vi "Tube Select.vi"(8 "error in (no error)":errorcluster) -> (0 "error out":errorcluster, 1 "Close":bool, 2 "Load":bool, 3 "SelectedTube":i32)   [LabVIEW 2023]
panel:
  in  "Close":bool
  in  "TubeSel":T1
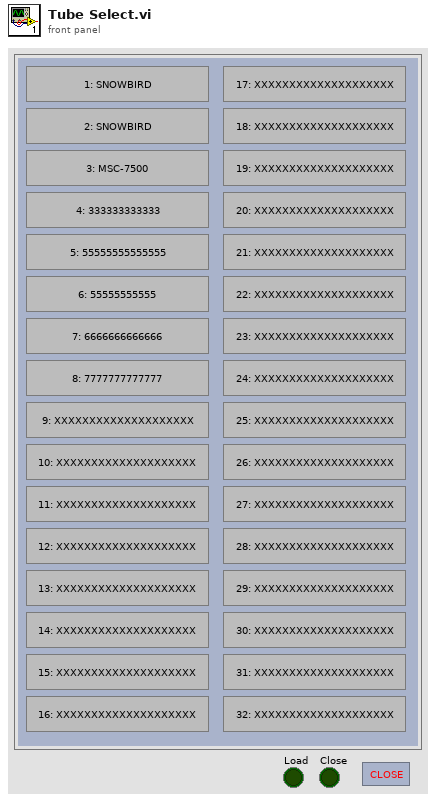
[diagram p1: front panel]
types:
  T1 = cluster{"OK Button 1":bool, "OK Button 2":bool, "OK Button 3":bool, "OK Button 4":bool, "OK Button 5":bool, "OK Button 6":bool, "OK Button 7":bool, "OK Button 8":bool, "OK Button 9":bool, "OK Button 10":bool, "OK Button 11":bool, "OK Button 12":bool, "OK Button 13":bool, "OK Button 14":bool, "OK Button 15":bool, "OK Button 16":bool, "OK Button 17":bool, "OK Button 18":bool, "OK Button 19":bool, "OK Button 20":bool, "OK Button 21":bool, "OK Button 22":bool, "OK Button 23":bool, "OK Button 24":bool, "OK Button 25":bool, "OK Button 26":bool, "OK Button 27":bool, "OK Button 28":bool, "OK Button 29":bool, "OK Button 30":bool, "OK Button 31":bool, "OK Button 32":bool}
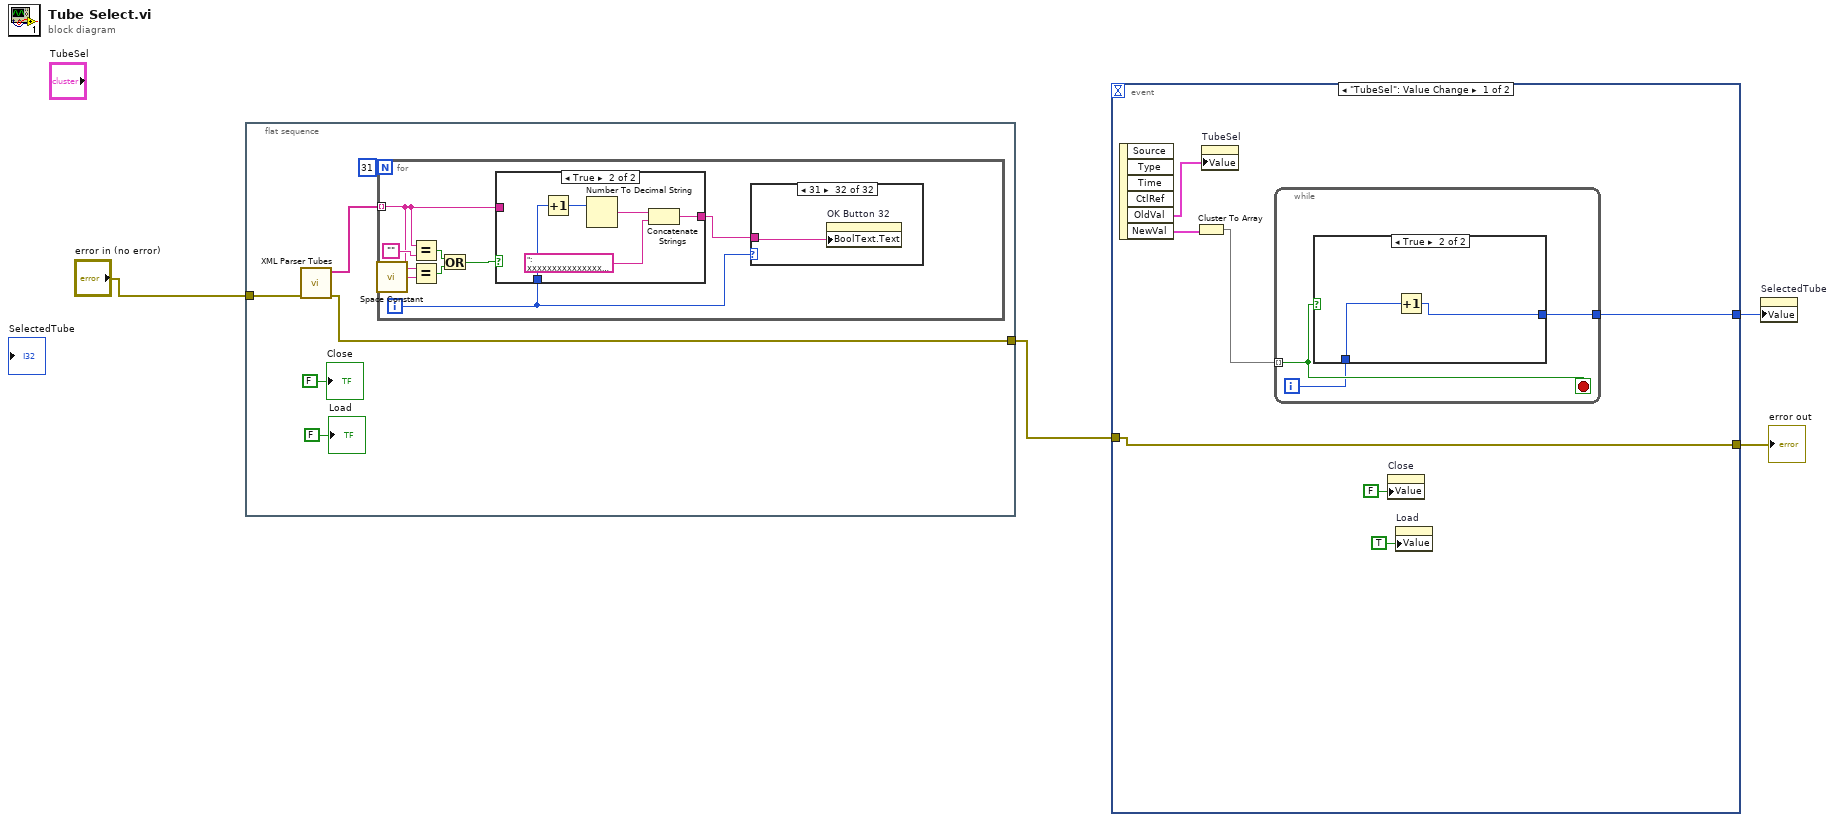
[diagram p0: block diagram]
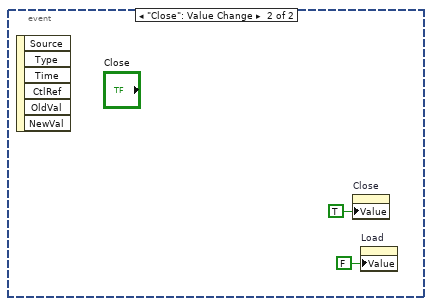
[diagram p3: hidden frame]
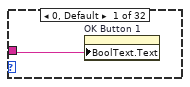
[diagram p4: hidden frame]
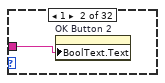
[diagram p5: hidden frame]
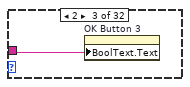
[diagram p6: hidden frame]
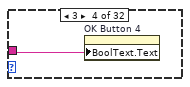
[diagram p7: hidden frame]
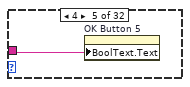
[diagram p8: hidden frame]
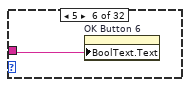
[diagram p9: hidden frame]
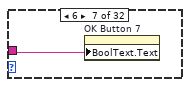
[diagram p10: hidden frame]
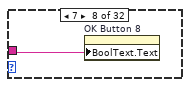
[diagram p11: hidden frame]
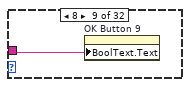
[diagram p12: hidden frame]
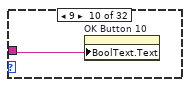
[diagram p13: hidden frame]
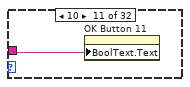
[diagram p14: hidden frame]
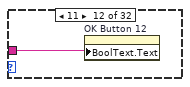
[diagram p15: hidden frame]
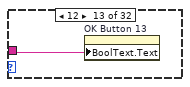
[diagram p16: hidden frame]
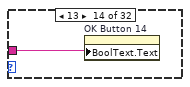
[diagram p17: hidden frame]
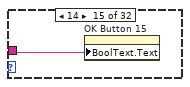
[diagram p18: hidden frame]
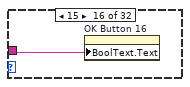
[diagram p19: hidden frame]
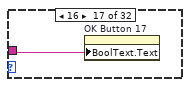
[diagram p20: hidden frame]
diagram:
  n1 = flat-sequence {
    tunnel: "error in (no error)" -> [w8]
    tunnel: [w7] -> w2
    frame #0 {
      n2 = call "XML Parser Tubes.vi"("error in (no error)"=w8) -> ("error out"=w7:errorcluster, "output array"=w10:string[])  [unwired: 9 in]
      n3 = for {
        N: 31 -> [_]
        tunnel: w10 -> [w13] mode=indexing
        i -> [w12]
        n4 = call <vilib>:"Space Constant.vi"() -> ("String"=w17:string)
        n5 = Equal?(x=w13, y="") -> (x = y?=w16:bool)
        n6 = Equal?(x=w13, y=w17) -> (x = y?=w15:bool)
        n7 = Or(x=w16, y=w15) -> (x .or. y?=w14:bool)
        n8 = case shown="True" w14 {
          tunnel: w13 -> [w54 _]
          tunnel: w12 -> [w51 w57]
          tunnel: [w53 w59] -> w11
          frame False {
            n9 = Increment(x=w51) -> (x+1=w52:i32)
            n10 = Number To Decimal String(number=w52) -> (decimal integer string=w56:string)  [unwired: 1 in]
            n11 = Concatenate Strings(w56, ": ", w54) -> (w53:string)
          }
          frame True {
            n12 = Increment(x=w57) -> (x+1=w58:i32)
            n13 = Number To Decimal String(number=w58) -> (decimal integer string=w61:string)  [unwired: 1 in]
            n14 = Concatenate Strings(w61, ": XXXXXXXXXXXXXXXXXXXX") -> (w59:string)
          }
        }
        n15 = case shown="31" w12 {
          tunnel: w11 -> [w19 w20 w21 w22 w23 w24 w25 w26 w27 w28 w29 w30 w31 w32 w33 w34 w35 w36 w37 w38 w39 w40 w41 w42 w43 w44 w45 w46 w47 w48 w49 w50]
          frame 0, Default {
            n16 = property on="OK Button 1" class="Bool (strict)"("BoolText.Text"=w19) -> ()  [unwired: 2 in, 2 out]
          }
          frame 1 {
            n17 = property on="OK Button 2" class="Bool (strict)"("BoolText.Text"=w20) -> ()  [unwired: 2 in, 2 out]
          }
          frame 2 {
            n18 = property on="OK Button 3" class="Bool (strict)"("BoolText.Text"=w21) -> ()  [unwired: 2 in, 2 out]
          }
          frame 3 {
            n19 = property on="OK Button 4" class="Bool (strict)"("BoolText.Text"=w22) -> ()  [unwired: 2 in, 2 out]
          }
          frame 4 {
            n20 = property on="OK Button 5" class="Bool (strict)"("BoolText.Text"=w23) -> ()  [unwired: 2 in, 2 out]
          }
          frame 5 {
            n21 = property on="OK Button 6" class="Bool (strict)"("BoolText.Text"=w24) -> ()  [unwired: 2 in, 2 out]
          }
          frame 6 {
            n22 = property on="OK Button 7" class="Bool (strict)"("BoolText.Text"=w25) -> ()  [unwired: 2 in, 2 out]
          }
          frame 7 {
            n23 = property on="OK Button 8" class="Bool (strict)"("BoolText.Text"=w26) -> ()  [unwired: 2 in, 2 out]
          }
          frame 8 {
            n24 = property on="OK Button 9" class="Bool (strict)"("BoolText.Text"=w27) -> ()  [unwired: 2 in, 2 out]
          }
          frame 9 {
            n25 = property on="OK Button 10" class="Bool (strict)"("BoolText.Text"=w28) -> ()  [unwired: 2 in, 2 out]
          }
          frame 10 {
            n26 = property on="OK Button 11" class="Bool (strict)"("BoolText.Text"=w29) -> ()  [unwired: 2 in, 2 out]
          }
          frame 11 {
            n27 = property on="OK Button 12" class="Bool (strict)"("BoolText.Text"=w30) -> ()  [unwired: 2 in, 2 out]
          }
          frame 12 {
            n28 = property on="OK Button 13" class="Bool (strict)"("BoolText.Text"=w31) -> ()  [unwired: 2 in, 2 out]
          }
          frame 13 {
            n29 = property on="OK Button 14" class="Bool (strict)"("BoolText.Text"=w32) -> ()  [unwired: 2 in, 2 out]
          }
          frame 14 {
            n30 = property on="OK Button 15" class="Bool (strict)"("BoolText.Text"=w33) -> ()  [unwired: 2 in, 2 out]
          }
          frame 15 {
            n31 = property on="OK Button 16" class="Bool (strict)"("BoolText.Text"=w34) -> ()  [unwired: 2 in, 2 out]
          }
          frame 16 {
            n32 = property on="OK Button 17" class="Bool (strict)"("BoolText.Text"=w35) -> ()  [unwired: 2 in, 2 out]
          }
          frame 17 {
            n33 = property on="OK Button 18" class="Bool (strict)"("BoolText.Text"=w36) -> ()  [unwired: 2 in, 2 out]
          }
          frame 18 {
            n34 = property on="OK Button 19" class="Bool (strict)"("BoolText.Text"=w37) -> ()  [unwired: 2 in, 2 out]
          }
          frame 19 {
            n35 = property on="OK Button 20" class="Bool (strict)"("BoolText.Text"=w38) -> ()  [unwired: 2 in, 2 out]
          }
          frame 20 {
            n36 = property on="OK Button 21" class="Bool (strict)"("BoolText.Text"=w39) -> ()  [unwired: 2 in, 2 out]
          }
          frame 21 {
            n37 = property on="OK Button 22" class="Bool (strict)"("BoolText.Text"=w40) -> ()  [unwired: 2 in, 2 out]
          }
          frame 22 {
            n38 = property on="OK Button 23" class="Bool (strict)"("BoolText.Text"=w41) -> ()  [unwired: 2 in, 2 out]
          }
          frame 23 {
            n39 = property on="OK Button 24" class="Bool (strict)"("BoolText.Text"=w42) -> ()  [unwired: 2 in, 2 out]
          }
          frame 24 {
            n40 = property on="OK Button 25" class="Bool (strict)"("BoolText.Text"=w43) -> ()  [unwired: 2 in, 2 out]
          }
          frame 25 {
            n41 = property on="OK Button 26" class="Bool (strict)"("BoolText.Text"=w44) -> ()  [unwired: 2 in, 2 out]
          }
          frame 26 {
            n42 = property on="OK Button 27" class="Bool (strict)"("BoolText.Text"=w45) -> ()  [unwired: 2 in, 2 out]
          }
          frame 27 {
            n43 = property on="OK Button 28" class="Bool (strict)"("BoolText.Text"=w46) -> ()  [unwired: 2 in, 2 out]
          }
          frame 28 {
            n44 = property on="OK Button 29" class="Bool (strict)"("BoolText.Text"=w47) -> ()  [unwired: 2 in, 2 out]
          }
          frame 29 {
            n45 = property on="OK Button 30" class="Bool (strict)"("BoolText.Text"=w48) -> ()  [unwired: 2 in, 2 out]
          }
          frame 30 {
            n46 = property on="OK Button 31" class="Bool (strict)"("BoolText.Text"=w49) -> ()  [unwired: 2 in, 2 out]
          }
          frame 31 {
            n47 = property on="OK Button 32" class="Bool (strict)"("BoolText.Text"=w50) -> ()  [unwired: 2 in, 2 out]
          }
        }
      }
      "Close" <- FALSE ("Close")
      "Load" <- FALSE ("Load")
    }
  }
  n48 = event shown="[0] \"TubeSel\": Value Change" {
    selector: _ -> [_ _]
    dyn-events: _ -> [_ _]
    timeout: _ -> [_ _]
    tunnel: [w66 _] -> w3
    tunnel: w2 -> [w63 _]
    tunnel: [w63 _] -> w1
    event "TubeSel": Value Change {
      n49 = event-data() -> ("OldVal"=w62:T1, "NewVal"=w68:T1)  [unwired: 1 in, 4 out]
      n50 = Cluster To Array(cluster=w68) -> (array=w67:bool[])
      n51 = property on="TubeSel" class="Clust (strict)"("Value"=w62) -> ()  [unwired: 2 in, 2 out]
      n52 = while {
        tunnel: w67 -> [w71] mode=indexing
        tunnel: [w69] -> w66
        i -> [w70]
        stop <- w71 stop-if-true
        n53 = case shown="True" w71 {
          tunnel: w70 -> [_ w73]
          tunnel: [_ w72] -> w69
          frame False {
          }
          frame True {
            n54 = Increment(x=w73) -> (x+1=w72:i32)
          }
        }
      }
      n55 = property on="Close" class="Bool (strict)"("Value"=FALSE ("Close")) -> ()  [unwired: 2 in, 2 out]
      n56 = property on="Load" class="Bool (strict)"("Value"=TRUE ("Load")) -> ()  [unwired: 2 in, 2 out]
    }
    event "Close": Value Change {
      n57 = event-data() -> ()  [unwired: 1 in, 6 out]
      n58 = property on="Close" class="Bool (strict)"("Value"=TRUE ("Close")) -> ()  [unwired: 2 in, 2 out]
      n59 = property on="Load" class="Bool (strict)"("Value"=FALSE ("Load")) -> ()  [unwired: 2 in, 2 out]
    }
  }
  "error out" <- w1
  n60 = property on="SelectedTube" class="DigNum (strict)"("Value"=w3) -> ()  [unwired: 2 in, 2 out]
